vi "WaveformDVR to gRPC .vi"(8 "error in (no error)":errorcluster, 10 "gRPC Waveform Enabled":bool, 11 "gRPC Waveform Monitor in":T3) -> (0 "error out":errorcluster, 2 "Waveform Monitor":T1, 3 "gRPC Waveform Monitor out":T3)   [LabVIEW 2021, in "CIFWaveformMonitorWrapper.lvlib"]
uses:
  CIFWaveformMonitorWrapper.lvlib
  CIFWaveformMonitor_client/RPC Messages/cif_waveformmonitor_Waveform.ctl
  CIFWaveformMonitor_client/CIFWaveformMonitor_client.lvlib
  CIFWaveformMonitor_client/RPC Messages/cif_waveformmonitor_Waveforms.ctl
  <vilib>/CIF Foundation/CIF Utilities/Time/Time_CIF_U.lvlib
  Typedef/WDT Array DVR.ctl
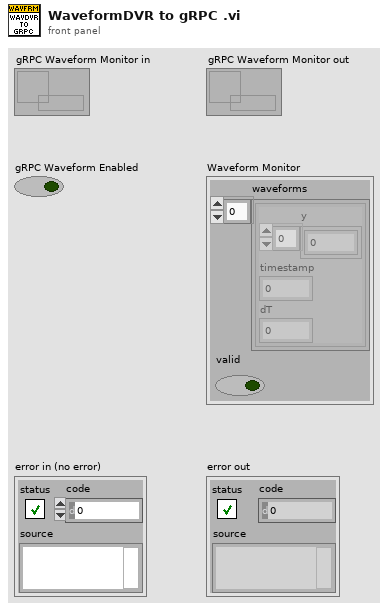
[diagram p1: front panel]
types:
  T1 = typedef "CIFWaveformMonitor_client.lvlib/cif_waveformmonitor_Waveforms.ctl" = cluster{"waveforms":T2[], "valid":bool}
  T2 = typedef "CIFWaveformMonitor_client.lvlib/cif_waveformmonitor_Waveform.ctl" = cluster{"y":dbl[], "timestamp":u64, "dT":dbl}
  T3 = typedef "CIFWaveformMonitorWrapper.lvlib/WDT Array DVR.ctl" = refnum<data-value>
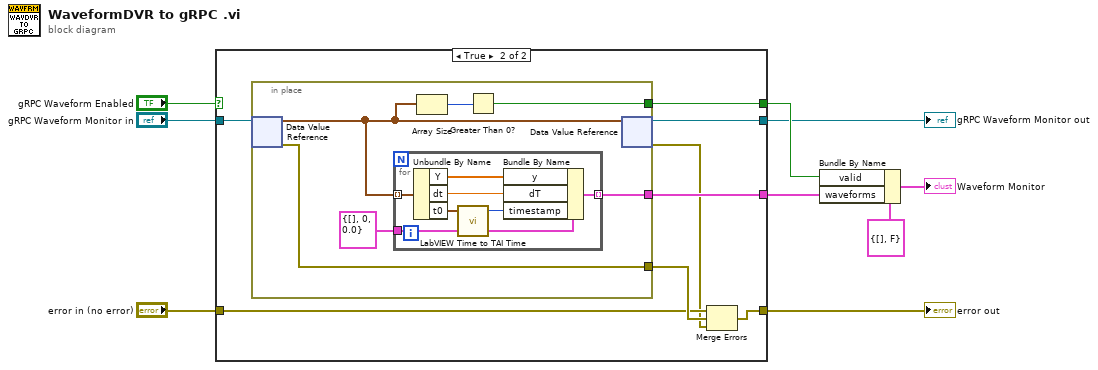
[diagram p0: block diagram]
diagram:
  n1 = case shown="True" "gRPC Waveform Enabled" {
    selector: "gRPC Waveform Enabled" -> [w12 _]
    tunnel: "gRPC Waveform Monitor in" -> [w10 w20]
    tunnel: [_ w19] -> w8
    tunnel: [w12 w18] -> w7
    tunnel: [w10 w17] -> w3
    tunnel: "error in (no error)" -> [w11 w15]
    tunnel: [w11 w13] -> w1
    frame False {
    }
    frame True {
      n2 = in-place {
        in-place-border: [w26] -> w19
        in-place-border: [w23] -> w18
        in-place-border: [w21] -> w16
        n3 = in-place-dvr #1(w20) -> (w25:waveform(dbl)[], w21:errorcluster)
        n4 = for {
          tunnel: w25 -> [w33] mode=indexing
          tunnel: T2 {"y"=[], "timestamp"=0, "dT"=0.0} ("cif_waveformmonitor_Waveform") -> [w32]
          tunnel: [w29] -> w26 mode=indexing
          n5 = Unbundle By Name(w33) -> ("Y"=w31:dbl[], "dt"=w30:dbl, "t0"=w28:timestamp)
          n6 = call <vilib>:"LabVIEW Time to TAI Time.vi"("LabVIEW Time (s)"=w28) -> ("TAI Time (ns)"=w27:i64)  [unwired: 4 in]
          n7 = Bundle By Name(cluster=w32, "y"=w31, "dT"=w30, "timestamp"=w27) -> (w29:T2)
        }
        n8 = Array Size(array=w25) -> (size(s)=w24:i32)
        n9 = Greater Than 0?(x=w24) -> (x > 0?=w23:bool)
        n10 = in-place-dvr #1(w25) -> (w17:T3, w14:errorcluster)
      }
      n11 = Merge Errors(w15, w16, w14) -> (w13:errorcluster)
    }
  }
  "error out" <- w1
  "gRPC Waveform Monitor out" <- w3
  n12 = Bundle By Name(cluster=T1 {"waveforms"=[], "valid"=FALSE} ("Message Data"), "valid"=w7, "waveforms"=w8) -> (→"Waveform Monitor":T1)
